vi "Read Filter Error Limits.vi"(8 "error in (no error)":errorcluster, 11 "Frequency Measurement in":refnum<class "Frequency Measurement.lvclass">) -> (0 "error out":errorcluster, 2 "Filter Error Limits (+/- V)":dbl=0.06, 3 "Frequency Measurement out":refnum<class "Frequency Measurement.lvclass">)   [LabVIEW 2013, in "Frequency Measurement.lvlib" / "Frequency Measurement.lvclass"]
uses:
  Frequency Measurement.lvclass
  Frequency Measurement.lvclass/Frequency Measurement.ctl
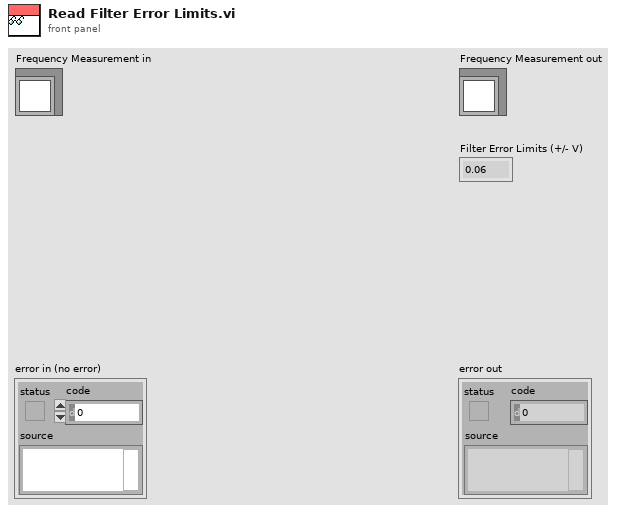
[diagram p1: front panel]
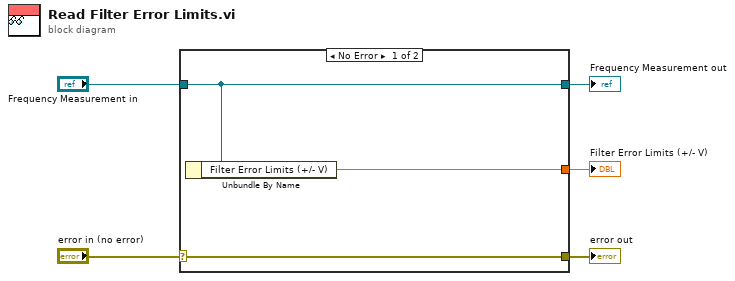
[diagram p0: block diagram]
diagram:
  n1 = case shown="No Error" "error in (no error)" {
    selector: "error in (no error)" -> [w8 w9]
    tunnel: [w8 w9] -> w4
    tunnel: [w7 w10] -> w2
    tunnel: "Frequency Measurement in" -> [w7 w10]
    tunnel: [w6 _] -> w1
    frame No Error {
      n2 = Unbundle By Name(w7) -> ("Filter Error Limits (+/- V)"=w6:dbl)
    }
    frame Error {
    }
  }
  "error out" <- w4
  "Frequency Measurement out" <- w2
  "Filter Error Limits (+/- V)" <- w1
